vi "Read Chassis Modules.vi"(8 "error in (no error)":errorcluster, 11 "Chassis in":refnum<class "Chassis.lvclass">) -> (0 "error out":errorcluster, 2 "Modules":refnum<class "Module.lvclass">[](array[class]), 3 "Chassis out":refnum<class "Chassis.lvclass">)   [LabVIEW 2016, in "SMI.lvlib" / "Chassis.lvclass"]
uses:
  Chassis.lvclass
  Module/Module.lvclass
  Chassis.lvclass/Chassis.ctl
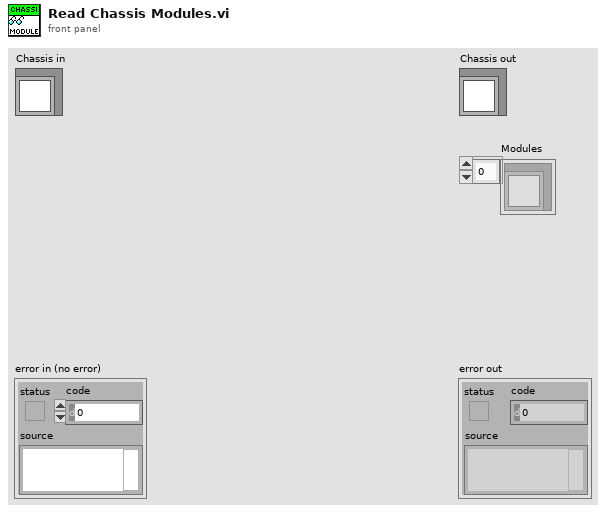
[diagram p1: front panel]
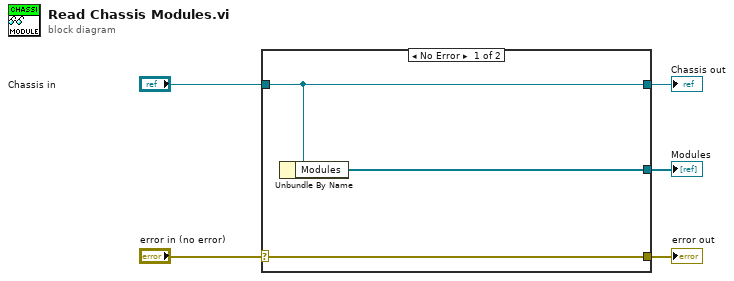
[diagram p0: block diagram]
diagram:
  n1 = case shown="No Error" "error in (no error)" {
    selector: "error in (no error)" -> [w8 w9]
    tunnel: [w8 w9] -> w4
    tunnel: [w7 w10] -> w2
    tunnel: "Chassis in" -> [w7 w10]
    tunnel: [w6 _] -> w1
    frame No Error {
      n2 = Unbundle By Name(w7) -> ("Modules"=w6:refnum<class "Module.lvclass">[])
    }
    frame Error {
    }
  }
  "error out" <- w4
  "Chassis out" <- w2
  "Modules" <- w1
